vi "MeasLeakRate07.vi"() -> ()   [LabVIEW 2011]
panel:
  out "XY Graph":cluster{"Value":dbl[], "Value":dbl[]}(graph)
  out "PT":dbl[][](array[numeric])
  in  "Control Valve local":bool
  in  "Exhaust Local":bool
  in  "Exhaust Close":bool
  in  "Exhaust Open":bool
  in  "Control Close":bool
  in  "Control Open":bool
  in  "reset":bool
  in  "# points to watch":i32=60
  out "leak rate (Torr/min)":string
  out "S20":dbl
  out "S11":dbl
  out "S10":dbl
  out "S01":dbl
  out "S00":dbl
  out "A11":dbl[](array[numeric])
  out "P":dbl
  in  "first":bool=TRUE
  out "A20":dbl[](array[numeric])
  out "A10":dbl[](array[numeric])
  out "A01":dbl[](array[numeric])
  out "A00":dbl[](array[numeric])
  in  "interval (s)":dbl=0.5
  in  "stop":bool
  out "P(Torr)":string
  # "Pressure control valve:"
  # "Exahaust valve:"
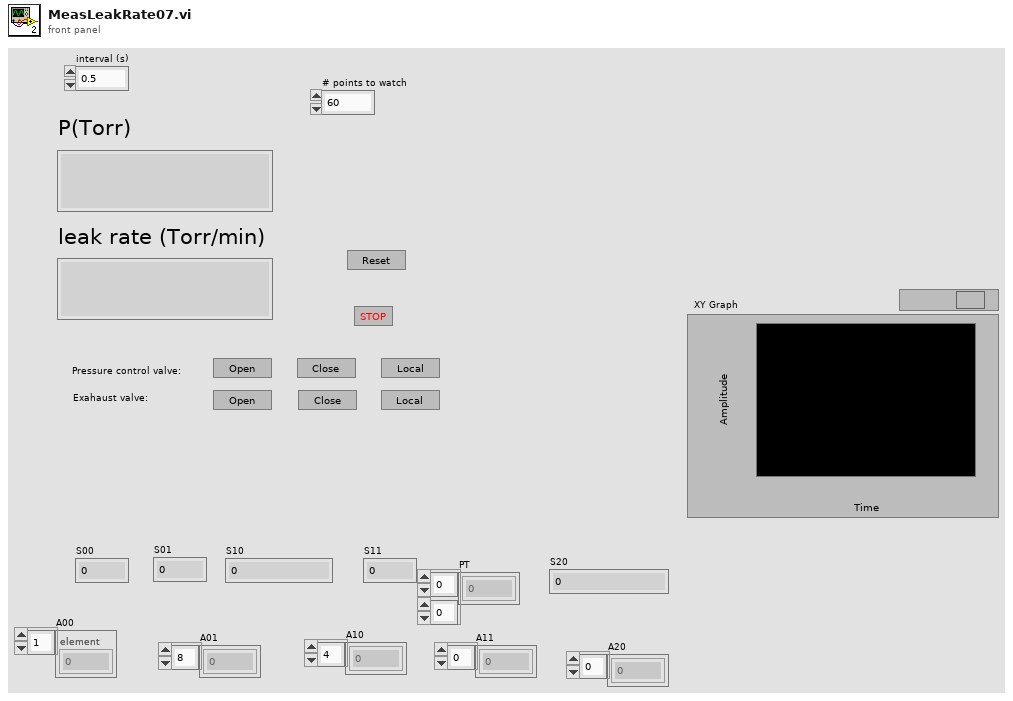
[diagram p1: front panel]
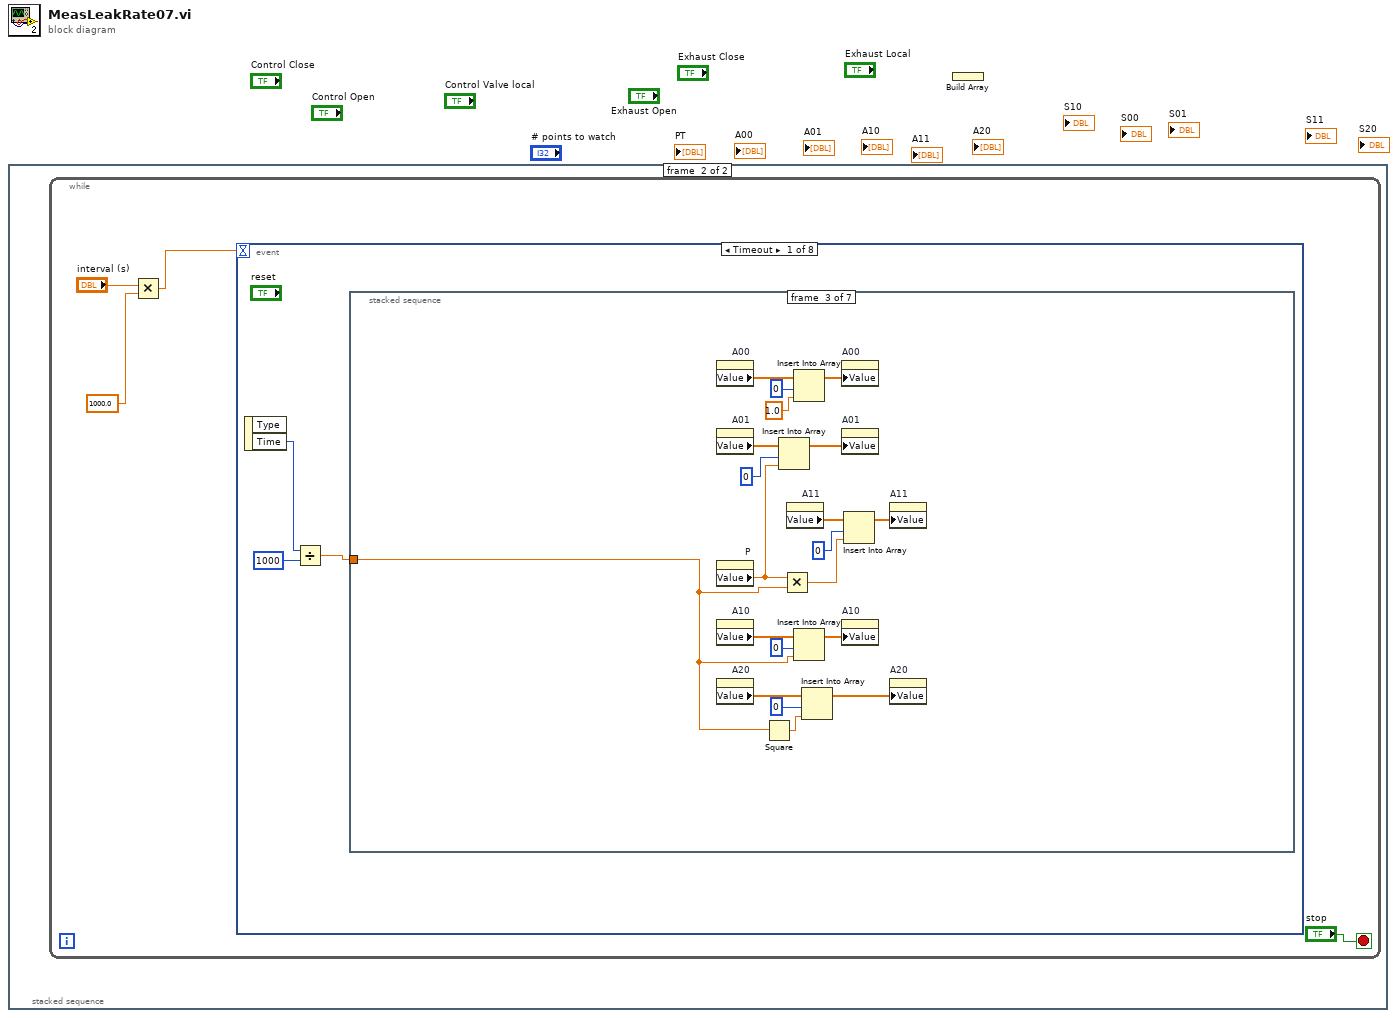
[diagram p0: block diagram]
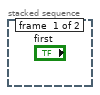
[diagram p2: hidden frame]
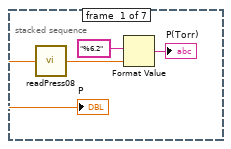
[diagram p3: hidden frame]
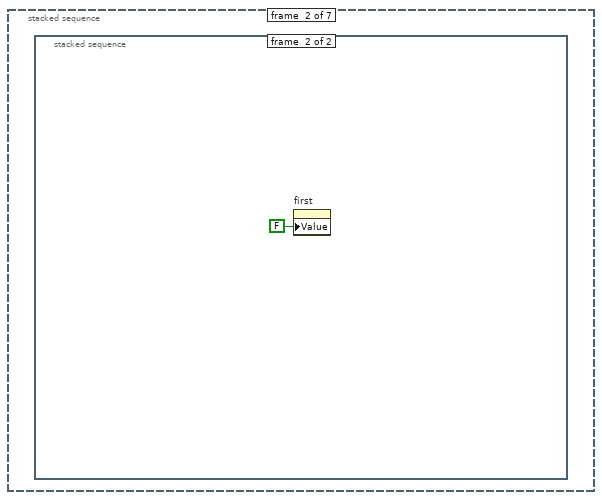
[diagram p4: hidden frame]
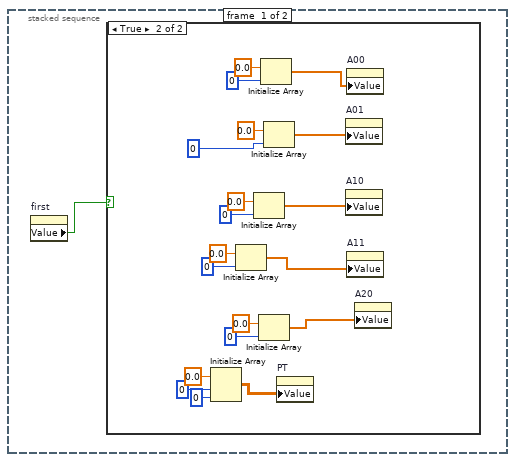
[diagram p5: hidden frame]
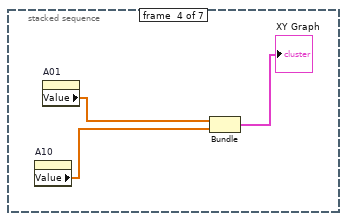
[diagram p7: hidden frame]
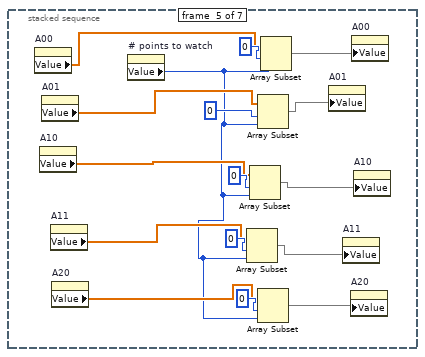
[diagram p8: hidden frame]
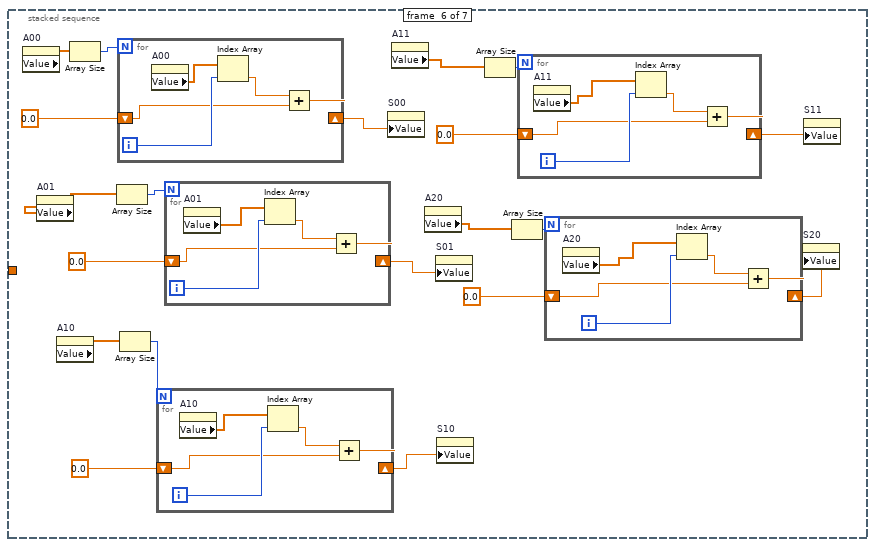
[diagram p9: hidden frame]
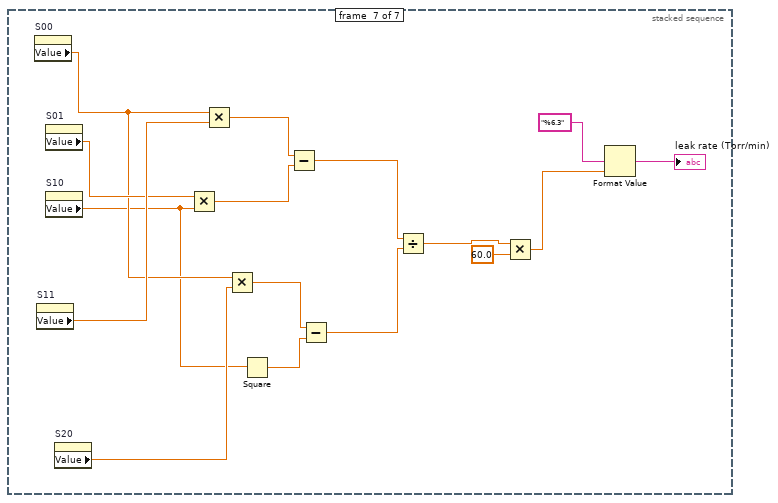
[diagram p10: hidden frame]
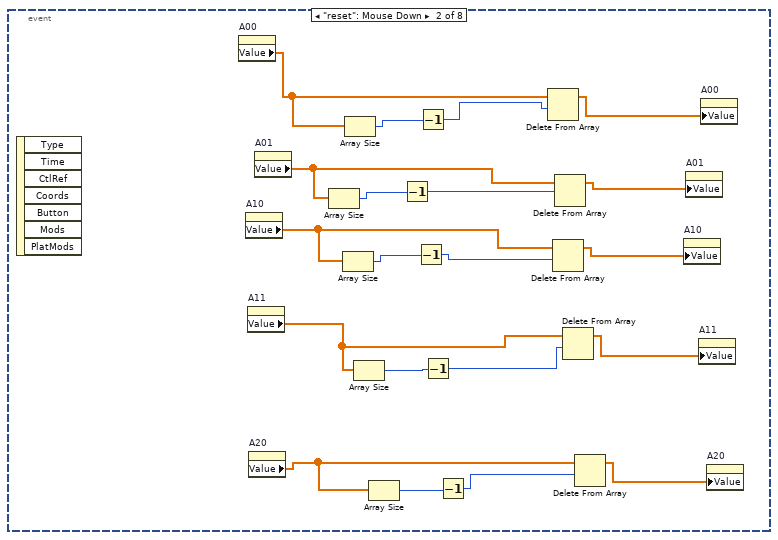
[diagram p11: hidden frame]
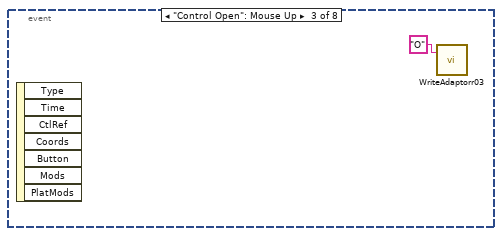
[diagram p12: hidden frame]
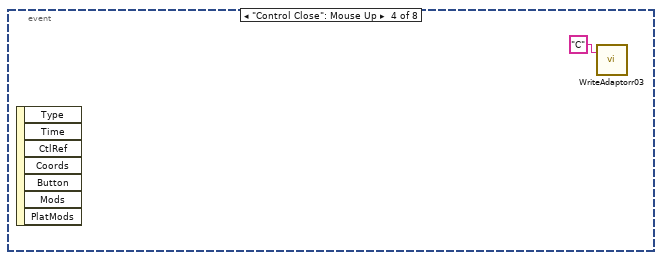
[diagram p13: hidden frame]
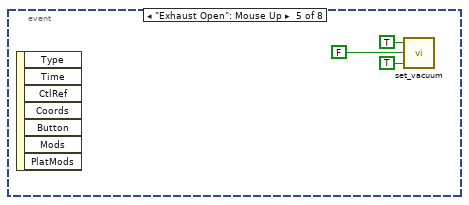
[diagram p14: hidden frame]
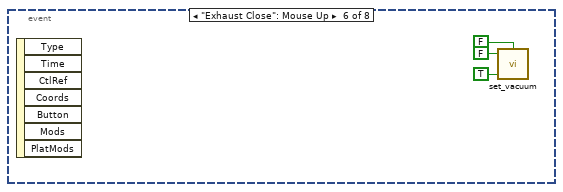
[diagram p15: hidden frame]
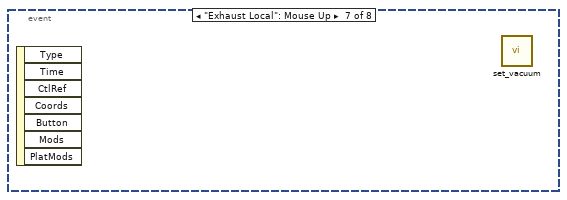
[diagram p16: hidden frame]
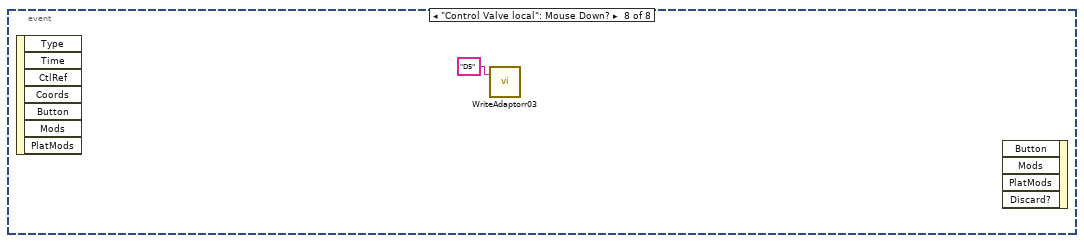
[diagram p17: hidden frame]
diagram:
  n1 = stacked-sequence {
    frame #0 {
    }
    frame #1 {
      n2 = while {
        stop <- "stop" stop-if-true
        n3 = Multiply(x="interval (s)", y=1000.0) -> (x*y=w2:dbl)
        n4 = event shown="[0] Timeout" {
          selector: _ -> [_ _ _ _ _ _ _ _]
          dyn-events: _ -> [_ _ _ _ _ _ _ _]
          timeout: w2 -> [_ _ _ _ _ _ _ _]
          event Timeout {
            n5 = event-data() -> ("Time"=w7:u32)  [unwired: 1 in, 1 out]
            n6 = Divide(x=w7, y=u32 1000) -> (x/y=w5:dbl)
            n7 = stacked-sequence {
              tunnel: w5 -> [_ _ w32 _ _ _ _]
              frame #0 {
                n8 = call "readPress08.vi"() -> ("P"=w9:dbl)
                "P" <- w9
                n9 = Format Value(format string="%6.2", value (0)=w9) -> (output string=→"P(Torr)":string)  [unwired: 1 in]
              }
              frame #1 {
                n10 = stacked-sequence {
                  frame #0 {
                    n11 = property on="first" class="Bool (strict)"() -> ("Value"=w11:bool)  [unwired: 2 in, 2 out]
                    n12 = case shown="True" w11 {
                      frame False {
                      }
                      frame True {
                        n13 = Initialize Array(0.0 ("element"), 0 ("dimension size"), 0 ("dimension size")) -> (w12:dbl[][])
                        n14 = Initialize Array(0.0 ("element"), 0 ("dimension size")) -> (w18:dbl[])
                        n15 = Initialize Array(0.0 ("element"), 0 ("dimension size")) -> (w19:dbl[])
                        n16 = Initialize Array(0.0 ("element"), 0 ("dimension size")) -> (w17:dbl[])
                        n17 = Initialize Array(0.0 ("element"), 0 ("dimension size")) -> (w16:dbl[])
                        n18 = Initialize Array(0.0 ("element"), 0 ("dimension size")) -> (w20:dbl[])
                        n19 = property on="PT" class="Arr (strict)"("Value"=w12) -> ()  [unwired: 2 in, 2 out]
                        n20 = property on="A01" class="Arr (strict)"("Value"=w20) -> ()  [unwired: 2 in, 2 out]
                        n21 = property on="A10" class="Arr (strict)"("Value"=w19) -> ()  [unwired: 2 in, 2 out]
                        n22 = property on="A00" class="Arr (strict)"("Value"=w16) -> ()  [unwired: 2 in, 2 out]
                        n23 = property on="A11" class="Arr (strict)"("Value"=w18) -> ()  [unwired: 2 in, 2 out]
                        n24 = property on="A20" class="Arr (strict)"("Value"=w17) -> ()  [unwired: 2 in, 2 out]
                      }
                    }
                  }
                  frame #1 {
                    n25 = property on="first" class="Bool (strict)"("Value"=FALSE ("first")) -> ()  [unwired: 2 in, 2 out]
                  }
                }
              }
              frame #2 {
                n26 = property on="A00" class="Arr (strict)"() -> ("Value"=w49:dbl[])  [unwired: 2 in, 2 out]
                n27 = property on="A01" class="Arr (strict)"() -> ("Value"=w47:dbl[])  [unwired: 2 in, 2 out]
                n28 = property on="P" class="DigNum (strict)"() -> ("Value"=w34:dbl)  [unwired: 2 in, 2 out]
                n29 = property on="A10" class="Arr (strict)"() -> ("Value"=w46:dbl[])  [unwired: 2 in, 2 out]
                n30 = property on="A20" class="Arr (strict)"() -> ("Value"=w44:dbl[])  [unwired: 2 in, 2 out]
                n31 = Square(x=w32) -> (x^2=w42:dbl)
                n32 = Insert Into Array(array=w47, index=0, new element=w34) -> (w35:dbl[])
                n33 = Multiply(x=w34, y=w32) -> (x*y=w40:dbl)
                n34 = property on="A11" class="Arr (strict)"() -> ("Value"=w41:dbl[])  [unwired: 2 in, 2 out]
                n35 = Insert Into Array(array=w49, index=0, new element=1.0 ("new element/subarray")) -> (w38:dbl[])
                n36 = Insert Into Array(array=w46, index=0, new element=w32) -> (w33:dbl[])
                n37 = Insert Into Array(array=w44, index=0, new element=w42) -> (w37:dbl[])
                n38 = property on="A00" class="Arr (strict)"("Value"=w38) -> ()  [unwired: 2 in, 2 out]
                n39 = property on="A01" class="Arr (strict)"("Value"=w35) -> ()  [unwired: 2 in, 2 out]
                n40 = property on="A10" class="Arr (strict)"("Value"=w33) -> ()  [unwired: 2 in, 2 out]
                n41 = Insert Into Array(array=w41, index=0, new element=w40) -> (w36:dbl[])
                n42 = property on="A11" class="Arr (strict)"("Value"=w36) -> ()  [unwired: 2 in, 2 out]
                n43 = property on="A20" class="Arr (strict)"("Value"=w37) -> ()  [unwired: 2 in, 2 out]
              }
              frame #3 {
                n44 = property on="A10" class="Arr (strict)"() -> ("Value"=w53:dbl[])  [unwired: 2 in, 2 out]
                n45 = property on="A01" class="Arr (strict)"() -> ("Value"=w54:dbl[])  [unwired: 2 in, 2 out]
                n46 = Bundle("Value"=w54, "Value"=w53) -> (→"XY Graph":cluster{"Value":dbl[], "Value":dbl[]})  [unwired: 1 in]
              }
              frame #4 {
                n47 = property on="A00" class="Arr (strict)"() -> ("Value"=w67:dbl[])  [unwired: 2 in, 2 out]
                n48 = property on="A10" class="Arr (strict)"() -> ("Value"=w61:dbl[])  [unwired: 2 in, 2 out]
                n49 = property on="A01" class="Arr (strict)"() -> ("Value"=w62:dbl[])  [unwired: 2 in, 2 out]
                n50 = property on="A11" class="Arr (strict)"() -> ("Value"=w60:dbl[])  [unwired: 2 in, 2 out]
                n51 = property on="A20" class="Arr (strict)"() -> ("Value"=w69:dbl[])  [unwired: 2 in, 2 out]
                n52 = property on="# points to watch" class="DigNum (strict)"() -> ("Value"=w55:i32)  [unwired: 2 in, 2 out]
                n53 = Array Subset(array=w60, index=0, length=w55) -> (w57:dbl[])
                n54 = Array Subset(array=w61, index=0, length=w55) -> (w58:dbl[])
                n55 = Array Subset(array=w62, index=0, length=w55) -> (w59:dbl[])
                n56 = Array Subset(array=w69, index=0, length=w55) -> (w56:dbl[])
                n57 = Array Subset(array=w67, index=0, length=w55) -> (w66:dbl[])
                n58 = property on="A01" class="Arr (strict)"("Value"=w59) -> ()  [unwired: 2 in, 2 out]
                n59 = property on="A11" class="Arr (strict)"("Value"=w57) -> ()  [unwired: 2 in, 2 out]
                n60 = property on="A20" class="Arr (strict)"("Value"=w56) -> ()  [unwired: 2 in, 2 out]
                n61 = property on="A00" class="Arr (strict)"("Value"=w66) -> ()  [unwired: 2 in, 2 out]
                n62 = property on="A10" class="Arr (strict)"("Value"=w58) -> ()  [unwired: 2 in, 2 out]
              }
              frame #5 {
                n63 = property on="A00" class="Arr (strict)"() -> ("Value"=w89:dbl[])  [unwired: 2 in, 2 out]
                n64 = property on="A01" class="Arr (strict)"() -> ("Value"=w85:dbl[])  [unwired: 2 in, 2 out]
                n65 = property on="A10" class="Arr (strict)"() -> ("Value"=w82:dbl[])  [unwired: 2 in, 2 out]
                n66 = Array Size(array=w89) -> (size(s)=w90:i32)
                n67 = Array Size(array=w85) -> (size(s)=w87:i32)
                n68 = for {
                  N: w90 -> [_]
                  shift-right: [w111] -> w75
                  shift-left: 0.0 -> [w112]
                  i -> [w114]
                  n69 = property on="A00" class="Arr (strict)"() -> ("Value"=w115:dbl[])  [unwired: 2 in, 2 out]
                  n70 = Index Array(array=w115, index=w114) -> (element=w113:dbl)
                  n71 = Add(x=w113, y=w112) -> (x+y=w111:dbl)
                }
                n72 = Array Size(array=w82) -> (size(s)=w84:i32)
                n73 = for {
                  N: w84 -> [_]
                  shift-right: [w102] -> w74
                  shift-left: 0.0 -> [w103]
                  i -> [w105]
                  n74 = property on="A10" class="Arr (strict)"() -> ("Value"=w101:dbl[])  [unwired: 2 in, 2 out]
                  n75 = Index Array(array=w101, index=w105) -> (element=w104:dbl)
                  n76 = Add(x=w104, y=w103) -> (x+y=w102:dbl)
                }
                n77 = for {
                  N: w87 -> [_]
                  shift-right: [w107] -> w73
                  shift-left: 0.0 -> [w108]
                  i -> [w110]
                  n78 = property on="A01" class="Arr (strict)"() -> ("Value"=w106:dbl[])  [unwired: 2 in, 2 out]
                  n79 = Index Array(array=w106, index=w110) -> (element=w109:dbl)
                  n80 = Add(x=w109, y=w108) -> (x+y=w107:dbl)
                }
                n81 = property on="S00" class="DigNum (strict)"("Value"=w75) -> ()  [unwired: 2 in, 2 out]
                n82 = property on="A11" class="Arr (strict)"() -> ("Value"=w79:dbl[])  [unwired: 2 in, 2 out]
                n83 = property on="A20" class="Arr (strict)"() -> ("Value"=w76:dbl[])  [unwired: 2 in, 2 out]
                n84 = property on="S01" class="DigNum (strict)"("Value"=w73) -> ()  [unwired: 2 in, 2 out]
                n85 = property on="S10" class="DigNum (strict)"("Value"=w74) -> ()  [unwired: 2 in, 2 out]
                n86 = Array Size(array=w79) -> (size(s)=w81:i32)
                n87 = Array Size(array=w76) -> (size(s)=w78:i32)
                n88 = for {
                  N: w81 -> [_]
                  shift-right: [w97] -> w72
                  shift-left: 0.0 -> [w98]
                  i -> [w100]
                  n89 = property on="A11" class="Arr (strict)"() -> ("Value"=w96:dbl[])  [unwired: 2 in, 2 out]
                  n90 = Index Array(array=w96, index=w100) -> (element=w99:dbl)
                  n91 = Add(x=w99, y=w98) -> (x+y=w97:dbl)
                }
                n92 = for {
                  N: w78 -> [_]
                  shift-right: [w92] -> w71
                  shift-left: 0.0 -> [w93]
                  i -> [w95]
                  n93 = property on="A20" class="Arr (strict)"() -> ("Value"=w91:dbl[])  [unwired: 2 in, 2 out]
                  n94 = Index Array(array=w91, index=w95) -> (element=w94:dbl)
                  n95 = Add(x=w94, y=w93) -> (x+y=w92:dbl)
                }
                n96 = property on="S20" class="DigNum (strict)"("Value"=w71) -> ()  [unwired: 2 in, 2 out]
                n97 = property on="S11" class="DigNum (strict)"("Value"=w72) -> ()  [unwired: 2 in, 2 out]
              }
              frame #6 {
                n98 = property on="S00" class="DigNum (strict)"() -> ("Value"=w127:dbl)  [unwired: 2 in, 2 out]
                n99 = property on="S11" class="DigNum (strict)"() -> ("Value"=w131:dbl)  [unwired: 2 in, 2 out]
                n100 = property on="S01" class="DigNum (strict)"() -> ("Value"=w130:dbl)  [unwired: 2 in, 2 out]
                n101 = property on="S10" class="DigNum (strict)"() -> ("Value"=w125:dbl)  [unwired: 2 in, 2 out]
                n102 = property on="S20" class="DigNum (strict)"() -> ("Value"=w126:dbl)  [unwired: 2 in, 2 out]
                n103 = Multiply(x=w130, y=w125) -> (x*y=w128:dbl)
                n104 = Multiply(x=w127, y=w131) -> (x*y=w129:dbl)
                n105 = Multiply(x=w127, y=w126) -> (x*y=w124:dbl)
                n106 = Square(x=w125) -> (x^2=w123:dbl)
                n107 = Subtract(x=w129, y=w128) -> (x-y=w122:dbl)
                n108 = Subtract(x=w124, y=w123) -> (x-y=w121:dbl)
                n109 = Divide(x=w122, y=w121) -> (x/y=w120:dbl)
                n110 = Multiply(x=w120, y=60.0) -> (x*y=w116:dbl)
                n111 = Format Value(format string="%6.3", value (0)=w116) -> (output string=→"leak rate (Torr/min)":string)  [unwired: 1 in]
              }
            }
          }
          event "reset": Mouse Down {
            n112 = event-data() -> ()  [unwired: 1 in, 7 out]
            n113 = property on="A00" class="Arr (strict)"() -> ("Value"=w151:dbl[])  [unwired: 2 in, 2 out]
            n114 = property on="A10" class="Arr (strict)"() -> ("Value"=w144:dbl[])  [unwired: 2 in, 2 out]
            n115 = property on="A11" class="Arr (strict)"() -> ("Value"=w141:dbl[])  [unwired: 2 in, 2 out]
            n116 = property on="A20" class="Arr (strict)"() -> ("Value"=w138:dbl[])  [unwired: 2 in, 2 out]
            n117 = property on="A01" class="Arr (strict)"() -> ("Value"=w147:dbl[])  [unwired: 2 in, 2 out]
            n118 = Array Size(array=w147) -> (size(s)=w146:i32)
            n119 = Array Size(array=w144) -> (size(s)=w143:i32)
            n120 = Array Size(array=w151) -> (size(s)=w149:i32)
            n121 = Array Size(array=w141) -> (size(s)=w140:i32)
            n122 = Array Size(array=w138) -> (size(s)=w137:i32)
            n123 = Decrement(x=w146) -> (x-1=w145:i32)
            n124 = Decrement(x=w143) -> (x-1=w142:i32)
            n125 = Decrement(x=w149) -> (x-1=w148:i32)
            n126 = Decrement(x=w140) -> (x-1=w139:i32)
            n127 = Decrement(x=w137) -> (x-1=w136:i32)
            n128 = Delete From Array(array=w151, length=w148) -> (array with subset deleted=w150:dbl[])  [unwired: 1 in, 1 out]
            n129 = Delete From Array(array=w144, length=w142) -> (array with subset deleted=w134:dbl[])  [unwired: 1 in, 1 out]
            n130 = Delete From Array(array=w147, length=w145) -> (array with subset deleted=w135:dbl[])  [unwired: 1 in, 1 out]
            n131 = Delete From Array(array=w141, length=w139) -> (array with subset deleted=w133:dbl[])  [unwired: 1 in, 1 out]
            n132 = Delete From Array(array=w138, length=w136) -> (array with subset deleted=w132:dbl[])  [unwired: 1 in, 1 out]
            n133 = property on="A10" class="Arr (strict)"("Value"=w134) -> ()  [unwired: 2 in, 2 out]
            n134 = property on="A01" class="Arr (strict)"("Value"=w135) -> ()  [unwired: 2 in, 2 out]
            n135 = property on="A11" class="Arr (strict)"("Value"=w133) -> ()  [unwired: 2 in, 2 out]
            n136 = property on="A00" class="Arr (strict)"("Value"=w150) -> ()  [unwired: 2 in, 2 out]
            n137 = property on="A20" class="Arr (strict)"("Value"=w132) -> ()  [unwired: 2 in, 2 out]
          }
          event "Control Open": Mouse Up {
            n138 = event-data() -> ()  [unwired: 1 in, 7 out]
            n139 = call "WriteAdaptorr03.vi"("string to write"="O") -> ()  [unwired: 1 in, 1 out]
          }
          event "Control Close": Mouse Up {
            n140 = event-data() -> ()  [unwired: 1 in, 7 out]
            n141 = call "WriteAdaptorr03.vi"("string to write"="C") -> ()  [unwired: 1 in, 1 out]
          }
          event "Exhaust Open": Mouse Up {
            n142 = event-data() -> ()  [unwired: 1 in, 7 out]
            n143 = call "set_vacuum.vi"("Vac Remote"=TRUE, "Atm Exhaust"=FALSE, "Vac Exhaust"=TRUE) -> ()
          }
          event "Exhaust Close": Mouse Up {
            n144 = event-data() -> ()  [unwired: 1 in, 7 out]
            n145 = call "set_vacuum.vi"("Vac Remote"=TRUE, "Atm Exhaust"=FALSE, "Vac Exhaust"=FALSE) -> ()
          }
          event "Exhaust Local": Mouse Up {
            n146 = event-data() -> ()  [unwired: 1 in, 7 out]
            n147 = call "set_vacuum.vi"() -> ()  [unwired: 3 in]
          }
          event "Control Valve local": Mouse Down? {
            n148 = event-data() -> ()  [unwired: 1 in, 7 out]
            n149 = call "WriteAdaptorr03.vi"("string to write"="D5") -> ()  [unwired: 1 in, 1 out]
            n150 = event-data() -> ()  [unwired: 5 in, 1 out]
          }
        }
      }
    }
  }
  n151 = Build Array() -> ()  [unwired: 1 in, 1 out]
